vi "Read Contact Check Measurement.vi"(8 "error in (no error)":errorcluster, 10 "Source Measure Unit Channel (0: Channel A)":i32(ring) items=["Channel A", "Channel B"], 11 "VISA resource name":refnum<visa-resource-name>) -> (0 "error out":errorcluster, 1 "Low Side Resistance":dbl, 2 "High Side Resistance":dbl, 3 "VISA resource name out":refnum<visa-resource-name>, 5 "Test Result":string)   [LabVIEW 2015, in "Keithley 2600 Series.lvlib"]
doc: "Returns the contact check result.\n\n<b>Note:</b>\nThis VI is not available on the models 2604B, 2614B and 2634B."
uses:
  Keithley 2600 Series.lvlib
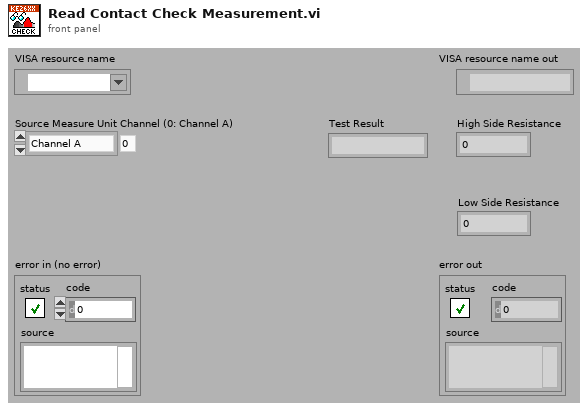
[diagram p1: front panel]
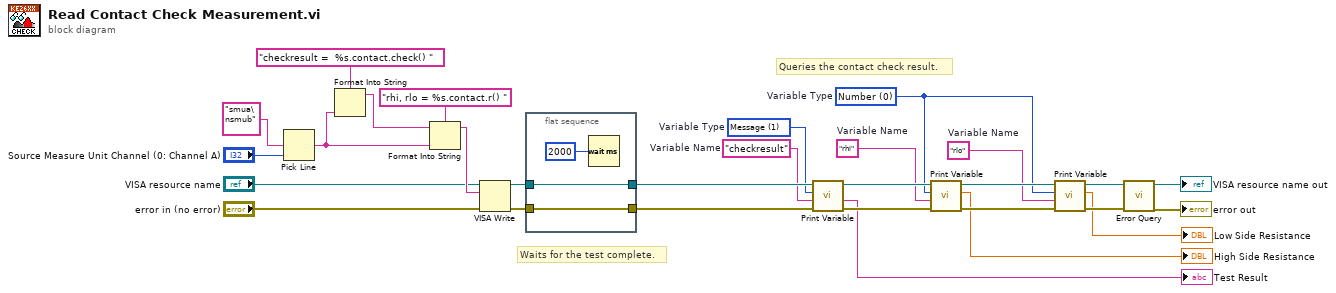
[diagram p0: block diagram]
diagram:
  w1 = 0 items=["Number", "Message"]  # Variable Type
  w2 = 1 items=["Number", "Message"]  # Variable Type
  w3 = "rlo"  # Variable Name
  w4 = "rhi"  # Variable Name
  w5 = "checkresult"  # Variable Name
  # "Waits for the test complete."
  # "Queries the contact check result."
  n1 = Pick Line(multi-line string="smua\nsmub", line index="Source Measure Unit Channel (0: Channel A)") -> (output string=w19:string)  [unwired: 1 in]
  n2 = Format Into String(format string="checkresult =  %s.contact.check() ", w19) -> (resulting string=w27:string)  [unwired: 2 in, 1 out]
  n3 = Format Into String(format string="rhi, rlo = %s.contact.r() ", initial string=w27, w19) -> (resulting string=w26:string)  [unwired: 1 in, 1 out]
  n4 = VISA Write(VISA resource name="VISA resource name", write buffer=w26, error in (no error)="error in (no error)") -> (VISA resource name out=w18:refnum<visa-resource-name>, error out=w17:errorcluster)  [unwired: 1 out]
  n5 = flat-sequence {
    tunnel: w18 -> [w31]
    tunnel: w17 -> [w32]
    tunnel: [w32] -> w15
    tunnel: [w31] -> w16
    frame #0 {
      n6 = Wait (ms)(milliseconds to wait=2000) -> ()  [unwired: 1 out]
    }
  }
  n7 = call "Print Variable.vi"("error in (no error)"=w15, "Variable Name"=w5, "Variable Type (0: Number)"=w2, "VISA resource name"=w16) -> ("error out"=w13:errorcluster, "Message"=→"Test Result":string, "VISA resource name out"=w14:refnum<visa-resource-name>)  [unwired: 4 in, 1 out]
  n8 = call "Print Variable.vi"("error in (no error)"=w13, "Variable Name"=w4, "Variable Type (0: Number)"=w1, "VISA resource name"=w14) -> ("error out"=w11:errorcluster, "Number"=→"High Side Resistance":dbl, "VISA resource name out"=w12:refnum<visa-resource-name>)  [unwired: 4 in, 1 out]
  n9 = call "Print Variable.vi"("error in (no error)"=w11, "Variable Name"=w3, "Variable Type (0: Number)"=w1, "VISA resource name"=w12) -> ("error out"=w9:errorcluster, "Number"=→"Low Side Resistance":dbl, "VISA resource name out"=w10:refnum<visa-resource-name>)  [unwired: 4 in, 1 out]
  n10 = call "Error Query.vi"("error in (no error)"=w9, "VISA resource name"=w10) -> ("error out"=→"error out":errorcluster, "VISA resource name out"=→"VISA resource name out":refnum<visa-resource-name>)  [unwired: 6 in, 2 out]
